vi "ws_get_targets.vi"() -> (0 "Error_info":string, 1 "Error?":bool, 2 "target_array":string[](array[string]))   [LabVIEW 2011]
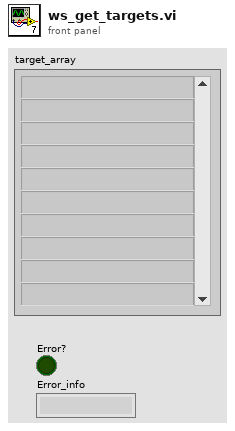
[diagram p1: front panel]
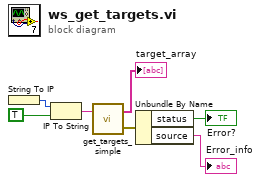
[diagram p0: block diagram]
diagram:
  n1 = String To IP() -> (0:w7:u32)  [unwired: 1 in]
  n2 = IP To String(1:TRUE ("dot notation? (F)"), 2:w7) -> (0:w3:string)
  n3 = call "get_targets_simple.vi"("Remote Server Address"=w3) -> ("error out"=w2:errorcluster, "Target Array"=→"target_array":string[])  [unwired: 1 in]
  n4 = Unbundle By Name(w2) -> ("status"=→"Error?":bool, "source"=→"Error_info":string)
